vi "2025_day4.vi"() -> ()   [LabVIEW 2025]
uses:
  <userlib>/_OpenG.lib/string/string.llb/openg_string.lvlib
panel:
  out "Task 1":i16
  out "Task 2":i16
  in  "Switch":bool caption="Ex. Data  vs.  User Data"
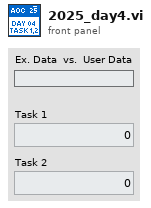
[diagram p1: front panel]
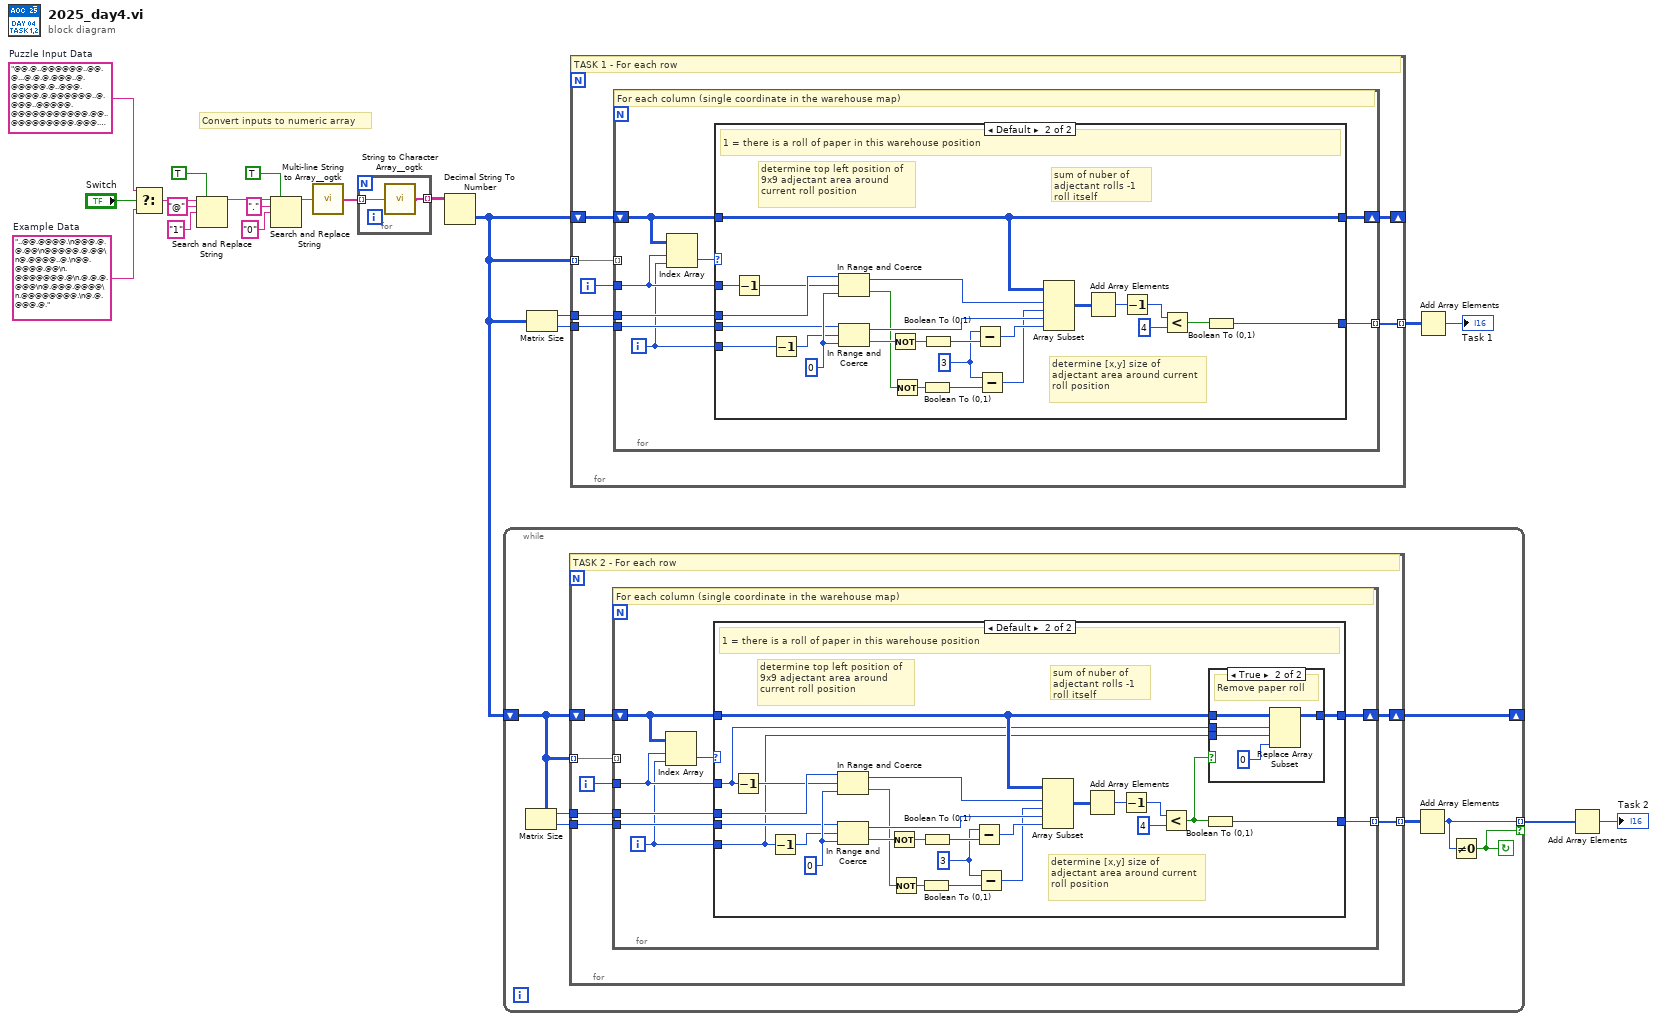
[diagram p0: block diagram]
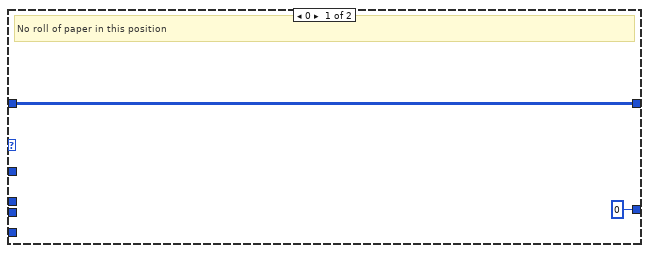
[diagram p2: hidden frame]
diagram:
  w19 = "@@.@..@@@@@@..@@.@...@.@.@.@@@..@.@@@@@.@..@@@.@@@@.@.@@@@@@..@.@@@..@@@@@.@@@@@@@@@@@.@@..@@@@@@@@@.@@@.@@@@@...@@@..@@@...@@@.@@@@@....@@@\n@.@@@.@@..@@@.@...@@..@.@@@@@@@@@@@@.@@@@....@@@.@@@@.@@.@..@@.@@@@@@@@@@@.@.@.@...@.@.@.@.@@..@.@@..@@@@@.@@@@@@..@@@@@...@..@@@@@.@..@@.@@\n@.@....@@@@.@@@@..@.@...@.@@@@@.@@@@@.@.@.@@@.@.@@@@@@@@...@@@@@@..@@..@@@@@@@@@@.@.@...@@@..@@.@@@..@@.@.@..@.@@@@@@.@@@@.@.@.@@.@@@.@@@.@@\n@@@@@@@@@@..@@.@@@@@@@@@@@@@@@@@.@@@@@....@.@......@.@.@.@..@@@.@.@@@.@...@@@@@@@@..@.@.@@..@@@@@@@@@.@@@@@@@@.@@@..@@.@.@@@@@..@@@.@@@@.@@.\n@@@.@..@@..@..@@..@@.@....@@@@..@@@@@....@.@@@.@@.@..@@@@.@@....@@.@@.@@.@@.@.@@@.@@@..@@..@.@..@@@@@@@@@@.@@@..@@.@@@.@@..@@@..@@@@@@@@.@@@\n@.@@@@@@.@@@@.@@@..@....@.@@@@@@@@@@@...@@.@@.@@@@@@..@@@@@@@...@.@@@@@@.@@@@@.@@@@@@@..@@@.@@@@@@@.@@@@@..@.@@..@@@.@.@@@@@@...@@.@@.@.@@..\n.@@@@.@.@..@@@@@.@@@@@.@@@@@.@.@@@.@@@@.@@@@@@..@@@@@@.@...@..@.@@@..@.@@.@@@@.@@.@@@..@@@..@@@@@.@@..@.@@@@.@.@@@.@..@..@@.@@@@...@@@.@@@@@\n..@.@@@@@@.@@@.@....@@@@@..@.@@@@..@@.@@@@.@..@@@@@@..@@.@@.@.@@@.@@.@@.@@@.@@@@@@.@..@@@@@@.@@@...@@@@@.@@@@@@@@....@.@@@@@@@@@@@..@@@.@@@@\n.@..@@.@@@.@@@@@.@@......@@@@@@@@.@@.@..@@..@@.@......@@..@@@@@..@@.@@...@..@@.@@@..@@.@@.@@@@@@@@@.@@@@@@.@@@.@@.@@.@...@@@@@@@.@@@@.@.@@@.\n@....@@@...@..@..@@@.@@.@@@@@@.@@@@@.@@@@.@@@@.@@@@@@@@@@..@@@@@@..@.@.@@..@.@@.@@..@.@@@.@.@.@@@@@.@.@..@@@@..@.@@..@@.@..@..@@.@....@@.@..\n@@..@@@@@@@@@@@.@.@@.@...@@@...@.@.@@@..@@.@@@@..@..@@@@@@@@@@@.@.@...@@.@@@@.@@@.@@...@@@@@.@.@.@@@.@@.@@.@.@@..@.@....@@.@.@@@@@@...@..@.@\n.@@@@..@@@@@@.@.@.@@.@@@.@@.@@.@@@@@.@.@.@.@@.@.@...@@@.@@..@.@..@@.@@.@@.@@..@@.@@@.@@.@.@@.@.@.@@@@@@@@.@..@@@@..@@.@@@.@.@.@@.@.@@..@@@@.\n@@@.@@@.@@@@@@@@@.@@@@..@@@.@@...@@.@...@@@.@.@@@...@@@.@@.@@@.@@@@@@@.@@@@.@.@@@@@@..@.@.@.@@...@@@@@@.@.@.@@@...@.@@@@@@@...@.@...@@@@@@@@\n@@@@@...@@@@.@@@..@@@@.@@@@.@.@...@.@@.@@@.@@@@.@..@@@...@.@@.@@@.@@.@.@.@@..@@@.@.@.@..@@..@.@@.@@.@..@@@.@..@.@@@@.@@@@.@@.@.@@@@@@@.@@.@@\n..@@...@@.@@.@@.@@@@@@@@@.@@.@@.@...@@@@@@@@@.@.@@@.....@@@@@@.@.@@..@..@@.......@.@@@@@@.@@@..@@@.@.@@@@@@@.@.@@..@@.@.@@@@.@@@.@@@@@@@..@@\n@@@.@@@.@@.@@..@.@.@.@@.@....@...@.@@.@@@.@@@@@..@@@@@@@@@.@@@@@@@@@@..@@...@.@@@@@@@.@@@.@@..@@@@@.@@.@..@..@@.@.@...@@.@.@@@@@@.@.@@@@@@.@\n@@@@.@@@..@@@.@.@.@@@@.@.@.@@.@@@@@@@..@@.@@@@@..@@@.@.@@@@.@@@..@@@@@@@...@@@@.@...@.@.@.@@@@@@@@@@@...@@@@@@@@@.@.@@@.@.@.@@@@@@@@@@@@@@.@\n...@@@@.@@.@@@@@@.@@@@@.@@@@@@@..@@@@@@.@...@..@@@....@@@@@@@..@@@@..@@.@@..@..@@@.@.@.@..@...@@@@@@@.@.@@@@@....@.@..@@@.@.@.@...@..@@@@@@@\n@@@@...@@...@.@.@@@@@.@@.@@..@...@@@@@@@@.@@@..@@.@@@@.@@@.@.@@..@..@@@@@@@@@...@@@.@@..@.@@@@.@@.@.@.@@@@@.@.@@@.@@@.@@@.@.@@@@@.@@@@.@@.@@\n@@.@@@.@@@@....@@@@@@@.@@@@@@.@@@@@....@.@@@@@.@@.@..@.@@.@@.@@.@@@@@@@.@@.@@...@..@.@@@.@@.@@@@.@@@@@@@.@.@.@@@@@.@.@..@@..@@@@.@@.@@@@@.@@\n@....@.@@.@@.@@..@.@@.@@@@@@@@@.@.@.@..@.@..@.@.@@.@@@@@.@@@.@..@@.@.@@@@@@@@..@@.@..@.@@@..@.@..@@@@.@@@@@@.@..@@@@@@.@@@@@...@..@.@@@...@.\n.@@@@.@@@.@.@@.@@@@@@...@@..@@.@..@@@.@.@..@@.@...@.@@@@.@@@.@..@@...@@...@@@@@@.@@.@@.....@@.@@@@@@@@@..@.@@@@@@@@.@@..@@.@.@@.@@@..@..@.@@\n@@@..@@@@......@@.@..@.@@.@@.@.@@@@@.@.....@@..@@.@@@@.@@@@@.@@.@@@@@@@@@@..@@@@@@@@@@@@@.@...@@@.@.@@@@@@@@@.@.@@@.@@.@@.@@@@.@@@@@@@@..@@@\n.@@@@@.@.@@@@@@@@.@.@@@...@@@.@@@...@@@@@.@.@.@@.@@..@@@@.@..@.@@@.@@@@@@@@@@@@.@@@..@.@.@@@@@.@@@.@@.@@.@@..@@@@@.@.@@@@.@@@@@...@@@@@@@@.@\n@.@.@@....@@@@@@.@..@@.@@.@@@@@@@@@.@@@@...@...@@..@@@@@.@@@@.@.@@.@@@@@.@@.@@....@@.@@.@@@@@@@.@@@@@.@@...@@.@@.@.@.@.@@.@@.@@.@..@@.@...@.\n@@....@..@@@@@@@@.@..@.@@.@@.@.@...@...@@..@@@@@@.@.@@.@@@@.@@.@.@@@@..@.@....@.@@..@@..@@@@@.@.@@@..@@@@@@.@@@@@@@.@.@@@@@@@@@@@@@@@@@@.@@.\n@@..@@.....@@@@@@@..@@@.....@@.@..@@@....@@@@@.@.@.@@.@..@@@@@@.@@@..@@..@@@....@.@.@@@@@...@@@@....@.@@@.@@.@@@@@.@.@..@@.@.@...@@.@..@@@@@\n@@@@..@..@.@.@@.@@@.@..@@.@@@@@@@..@@.@@..@@@.@@@@.@.@@@@@@@.@@..@@@@@@@.@@@@@@@.@@.@@..@@@@@@@@@..@..@@..@.@@.@.@.@@@@@.@@@@@@.@....@@..@@.\n@@....@@@.@.@..@@.@.@@.@.@@@...@.@@...@@@@@@.@@@@.@.@@@.@..@@@@..@@@@@@@@@@@.@@.@@@@@@@.@.@@@@.@.@@@@....@@..@@.@@..@.@@...@@..@..@.@@@@...@\n@@@@@@@@..@@.@@....@@@@.@@@.@@@@@@.@.@@..@@@@@@.@@@@.@@.@@@@.@@@.@.@@..@@@@@@@@@@@@...@..@.@..@@@.@.@@@..@@@.@.@@@@@@@@@@@@..@@@@.@.@@.@.@.@\n@@.@@@@..@@@..@.@.@.@@@.@.@@@@...@@@@@.@.@@...@@@@@..@.@@.@.@@@@.@.@@..@.@.@@@...@...@...@.@@@@@@..@@.@..@@.@.@..@@@@@@.@@@@@@@@@@@@@@@.@.@@\n@.@@@.@@@...@.@@@@@@@@@@@@..@@@@.@.@@....@@@.@.@@@@.@@..@@@.@@@@@..@.@@@@...@.@@..@@.@@.@@@@@..@@.@.....@@..@@..@@@.@.@.@@@@@@@@@.@@@..@@@.@\n..@.@@..@@..@@.@@..@.@@.@..@@..@@@@@..@@@@.@.@@.@@@@@@@.@@.@.@@@@@.@@.@@..@.@@@.@..@@@.@@.@.@@@@....@.@@@..@@..@.@@...@@@..@@..@@@@@@@@@@@.@\n@@.@@@@..@@@@@@.@@@..@.@@..@..@@@..@.@@@@@@@@..@.@@..@@@.@@...@@@.@@@@.@@.@@@@.@.@@@@.@@@.@@@@@.@@@@@.@.@@.....@@@@@..@@.@.@@@@.@@@@.@@@@@@@\n@@@@.@..@@@@@@@@..@@@..@@@@@@@@@.@@@..@@.@@.@..@@.@@@@.@@@@@@@@@@@@@..@@@..@@@@.@@@@@@@@@@@@@..@@.@.@.@..@.@.@..@.@@.@@@.@@@@.@.@@.....@....\n@.@..@@.@@@@.@@@.@@...@@.@@.@@@...@@..@@.@@@@.@..@@@@@@@@@@.@@@@@@@@@@@@@@..@.@.@.@@@@@@.@@@@...@@@@@@@@@..@@.@@.@@.@@@..@@@@@....@.@..@@@@.\n...@.@@@@@...@@@@@@@@@.@..@.@@..@.@@@@@.@.@@.@...@@@@@..@..@@@@@.@@@@@@@@@@@@....@@.@@.@@.@.@@@@.@@@@..@.@@@@@@@@@.@@@@..@@@@@@@@@@.@@@.@.@@\n@@@..@.@@@@@@@@@.@@@....@@@@@@@.@@@@@.....@@@..@@@@@.@@@@@@@@.@@@@@@.@@.@..@..@@@@@.@.@......@@@@@@@.@.@@.@@@@@@@@@.@@@@@@.@@@.@@@@.@.@.@.@.\n@..@@....@@.@.@@@@@@..@@...@@.@...@@.@.@....@@.@@@.@@...@@.@@.@.@@@@.@.@@@@@.@@.@.@@...@@.@@@@...@@@@@.@@..@.@@@@@..@@@@@@@.@@.@.@@@@@@@@@@@\n..@.@@@@@@.@.@@.@@..@@@....@.@@..@.@@.@.@@@@@@..@@@.@@.@@@.@@@@@...@@@@@.@.@@.@@@@..@.@@@.@.@@@.@@@.@@..@@@@@@@@..@@@@@@@@@..@.@.@@@@..@@@@.\n@@@@@.@.@@@@@.@@@@..@..@.@.@@@@.@@@@@@..@@@@@..@@@@...@@@..@@@.@@@.@@@@..@..@.@.@...@@@.@@@@.@...@@@.@@@....@@@@@@...@.@@@..@.@.@@@.@...@.@@\n@@@@@...@@@.@@.@@.@.@@.@@.@@@.@@@@@.@@..@@.@@@@@@@@@.@@.@@@.@@@.@@.@@.@@@@@..@.@@.@..@@...@...@@..@@.@@.@@.@@@@.@.@@@@.@@@.@@..@.@@.@..@@.@@\n..@@.@@..@....@@@..@.@.@@..@.@@.@.@@@.@@@.@.@.@@@@@...@.@@@.@@@@@..@.@@.@..@@@@.@@@@@@@@@.@@@@.@@.....@@@..@@@...@@@.@@@@@@@..@.@@@.@@@.@.@@\n..@@@@@..@@@.@.@@..@@@@@.@@@@@@@@@@.@@@@@.@@@..@..@@@.@@@.@.@@.@@@@@.@@@..@@@.@..@..@.@.@@.@.@@@@@@.@..@.@@@@@.@@@@@..@@.@@@@@..@@@@@@@.@@@@\n@.@@@.@.@@@..@@@@@...@.@@@@@.@@@@@@.@@@@..@.@@.@@.@.@@@@...@@@@@@@@.@@@@..@....@@@@@@.@.@@@..@.@.@.@@@.@.@@.@@.@@@@@..@@.@.@@@.@...@@@.@@.@@\n@@@@@..@@.@@@@@@@@@@@@@....@@@@@@@.@.@@@@.@@@@.@.@@@@@@@@.@.@@@.@@.@.@.@@.@.@..@@@@@@@@@@@@@.@...@@@@@.@@..@.@@@@@@@@.@@@.@@@@@@.@.@..@.@@@@\n@...@@.@@@@@@.@@@@@.@@@.@@@@@@.@@@@@@.@@.@...@@.@@@@..@@.@@@.@.@@@@@.@@@...@@@@@@@@@@@.@@@@.@..@..@@@@@@@@@..@@.@.@..@@@@@@@.@..@@@@..@.@.@.\n.@..@@...@.@.@@.@.@...@@@@@....@@@.@...@.@@.@@@.@..@.@..@.@.@@@.@@.@@@@@@@.@@.@.@.@@...@@@@@.@@@@@@@.@..@@.@.@.@.@..@..@@.@@.@.@.@@@.@.@@@@@\n@@@.@@@@.@@.@@@..@@.@@@@.@.@@.@.@.@@..@@@@.@.@@@@.@@..@@@...@.@@@@@@.@@@.@..@.@@@@@.@..@@...@.@@.@@@..@.@.@..@@@.@@@..@@@@@@.@@@.@@.@@@@@@@@\n@@@@..@.@@@@@@.....@@.@@@..@.@@.@.@@@@.@...@@@.@@@.@..@.@.@@@.@.@@@..@@@@@@@.@@.@@.@@@@@.@@....@@.@@.@@..@@@.@@@.@.@@@.@@@@@@@@.@@@.@....@@@\n@@@@@@.....@..@@@@@@@.@@.@@@@@.@.@@@@..@@@....@...@.@@..@@.@@...@.@.@.@@@.@.@@@@@..@.@@@@..@@@@@.@@@.@@.@@@..@@@@@..@@@.@@..@@@@.@@@...@.@@@\n@@@@@@..@.@@@@@@@@@.@@@@@.@@.@.@@@@@@@@@@@@@@.@..@@@@....@@@@.@.@.@@@.@@.@...@@@@@@@...@@@...@@.@@@@@@.@@@@@.@@...@.@@@@@@@@.@@.@@@@@@@@.@@@\n@...@.@@@.@@@@@@..@@...@@@.@..@@.@@@@@.@...@..@@@.@@@@@.@.@@@@@.@@@@@@@@@@.@@.@....@@@@@..@@@..@@@@..@@...@@@@.@@@@@.@.@..@@@@.@@.@@..@@@.@@\n@.@@..@@@.@.@.@@.@@.@@@@@@@.@@.@.@@.@@.@.@...@@@@@.@..@@@@.@..@.@@.@.@@@@...@@...@@@@.@...@.@.@@@..@@..@@@....@@@@.@..@..@@@@.@@@@@@.@.@@.@.\n@@@@.@.@@@@..@.@@....@@@..@@@@@.@@..@..@@.@@..@@.@@...@...@@@@..@@...@@@@@@@@@@..@@@.@@@.@@@@@@.@@..@@@.@@@.@@@.@.@.@@.@.@.@@.@@@@@@..@..@.@\n@@@@.@.@@.@@.@...@@@@@@@.@.@@@@...@@@.@@@@@.@@@@@.@.@@@@@@@..@@.@@..@@.@@@@@@..@@@.@@@.@....@@@@.@....@@@@@@.@.@@@@@@@.@.@@..@@@@@@@@..@@@@@\n@..@...@@@@..@.@...@@@@.@@@..@@@..@@.@@...@@@@@@@@..@@@.@@@@@@@@@@@...@...@@@@.@.@@@@@@@.@.@.@@....@@@@.@.@@@@..@.@@@..@..@.@@@.@.@...@@@.@.\n..@@@.@.@@@@.@.@@@@@@@@@@@@@.@.@@@@@@@@@@@.@@@@@@.@@@@@.@@.@@@.@@@.@@@@.@.@@.@@..@@..@.@@@.@@@@@@@.@@.@@@...@@.@@@@@...@..@@@@@@.@@@@@.@@@@@\n@@@@@@@..@@..@@.@@@.@@@.@....@@@@@.@@@.@@@@.@..@@@@.@@.@@@.@@@@@.@@@@@@@@@..@@@@@@@...@.....@@.@@@@@@@..@.@.@.@@@.@@.@@@@..@@.@@@.@.@@.@@..@\n@@.@@...@@@@@@.@@@@.@.@.@.@.@@.@...@@@@.@.@@@@....@@.@.@@@@@@@.@@@...@..@@.@..@@@.@.@.@.@.@.@@..@@@@@.@@..@@.@..@@@.@@@.@.@...@.@@@.@@@@.@@@\n.@.@.@.@@.@@.@..@@@.@.@@@.@@@...@.@...@@@...@@.@@@.@@@@@@.@.@...@...@@....@@....@.@@...@@.@@@@.@.@@@@@@@@@.@@@@@.@@@@@..@@.@@@@@.@@@@@@@.@@@\n@@@.@.@..@@@@@@@@@@@@@.@@@.@@@@@@.@@@..@.@...@@@@@.@.@@.@@.@......@.@.@@.@@@@.@@@...@@@@@@@@@@.@.@@.@.@@@@@@@@.@@@@@..@@.@@.@@@.@.@@.@.@@.@.\n@@..@@@@@.@.@.@@@@.@@.@.@@...@.@@..@@@@@@@@@@.@@@@@.@@@..@.@.@@@@@.@.@@@....@.@@.@..@..@@..@@.@@@..@@...@@.@.@@@.@@..@@@@@@@..@@@@@@.@.@.@@@\n@..@@.@.@.@@.@@@...@@.@..@@@@.@.@@@...@..@@.@.@.@@@..@@@@.@@@@@@@@.@@@@@@@..@.@@@@@@.@@@@...@@@@.@@.@@.@.@..@.@@..@.@.@@@.@@.@@@.@.@..@@@@@@\n@@..@.@.@..@.@@@@.@@@@@.@...@@@.@....@..@@@@@@@@@.@@..@.@.@@@@@@.@@..@@@@.@.@.@...@@..@@..@@@@@@@...@@@@@.@.@...@@@@...@@..@@@..@@..@@.@@..@\n@@@@....@..@@@...@@.@@@@@.@@@@.@...@@@@@@@@@@...@.@.@@@@.@@.@@@@@..@@@@@.@.@..@..@@@@.@@.@@@@@@@@.@@@@@@.....@@@@@...@.@....@@@@@@@@@@@@@..@\n@@.@@@.@@..@@.@@@..@@@.@@..@..@...@@@@@@@..@@@@@@@.@@.@@@@@.@@.@@@@.@.@@@..@@@.@..@@@@@..@.@@@@..@@@@...@@@@@@@..@..@.@@@..@.@@@@@@@@@@.@@.@\n@@@@....@@@.@@@@..@@@@@@..@@.@@.@@.@@@@@..@.@@..@..@@.@@@.@..@@@.@@@@@@.@@@.@@@..@@@@..@@@.@@@@..@@.@@@@..@@@..@@.@@@..@@@@@@@@@...@@@.@@@@@\n@@.@.@@@.@@@@..@@.@@@.@@@@.@.@@.@....@.@@@@.@@@@@@.@@@@@..@@@.@@@@@@.@@@.@@@@@@@.@@@@@@@@@@@.@.@@@.@....@.@..@.@@@..@.@...@@.@.@@@.@.@@@@@@@\n@@@@@@@.@.@@@.@@.@@.@...@@.@@.@@@@..@.@@.@@@.@..@@.@..@..@.@..@@@@@@.@.@...@@@@.@@@..@@@@..@@@.@@@@@@..@@@@@@@@.@@@@@@.@..@.@@@@@..@@@.@@@@@\n.@@.@.@@@..@@.@@.@.@@@...@@.@@@@@.@@@@@@..@@@.@.@@@.@@@....@...@@@.@.@@@.@@@@@@.@@@@..@.@.@.@.@@@@@.@@@@.@@@@.@@@...@@@@...@@.@.@@@..@@@.@@@\n...@.@.@@@.@@@@@.@@....@.@@@.@.@@.@...@@@.@.@@@@.@..@@.@@@@@@.@@@@@.@@@@@@@@.@@@@..@.@@....@@.@@@@@@..@..@@@@.@@..@.@@@@@@@@@@.@..@.@@@@@@@@\n@@.@..@@@@.@@@@@@.@@.@@@@@.@@.@.@@@..@@..@..@@.@.@@@@@.@@@@@@@@@.@@.@@..@.@@@@@@.@@@@@@.@@@.@@@.@@.@.@@.@@@@@@....@..@@@..@@@.@@@@.@@@@@@.@@\n@@@.@.@@@.@@.@.@.@@..@@@@.@.@@@.@.@...@..@..@..@.@@@.@@.@@@.@@@.@@@@@@@@@@..@@..@@.@....@@@.@.@@..@.@@.@.@@@@@@..@@.@@.@..@.@@....@.@.@@@.@@\n.@.@@.@..@..@@.@@.@@@@@@@@@@@@@..@.@@@@@@.@@@.@@@@@....@@..@@..@...@@..@.@.@@.@@@@.@@.@@@..@@@....@@@..@.@.@.@@@..@....@@.@@@@@.@@@....@@@@@\n@...@@.@..@@@@@@..@@@@.@@@...@@@..@@@.@@.@@@@.@..@@@@..@..@.....@@@.@@@.@@..@..@@@@.@.@@.@@.@@@@.@@.@.@.@...@@@.@@@.@..@@.@@..@@@.@...@@@@@@\n@.@@@.@@@.@...@@@@@@@@@@.@@@@@@.@.@..@....@@@...@@@.@@@@@..@@.@....@..@@.@.@..@@@@.@@@.@.@@@@@@@.@@@@@@@@@.@@@@@@.@@@@@@@.@..@@@@@@@@.@@..@.\n@@..@@@@.@@@@@.@@@.@.@@@.@@.@.@.@@@@@@@...@...@.@.@@.@@@@@@@.@.@...@@@@@@.@@.@@...@@@..@@@@@@@.@.@.@@..@....@@.@@.@@@@.@@@@@@@..@.@@....@.@.\n.@..@.@..@@@@...@..@@@.@@.@@@.@@@@.@.@@@@@@.@@@@@@@..@@@@.@..@@@.@@.@.@.@@.@@@@.@@@.@@.....@.@@@@@.@....@@@.....@@.@..@@@.@@@.@@..@.@@@@.@@.\n@@.@.@...@....@.@..@@.@@..@.@.@@@@.@.@@...@@@.@.@.@@..@@@.@@.@@.@@@.@@@@@...@@.@@@.@..@..@..@@@@@..@@@.@@..@@.@@@@..@@@.@@@@.@.@.@@.@@@@@@..\n.@@.@@.@.@..@..@@..@.@@.....@@@@@.@@@@@@.@..@..@@@@.@.@.@@@.@.@.@.@.@@...@@.@@.@.@@.@@@.@@@@@@.@.@@@@@@@@@.@.@@@@@..@@@@@.@.@@@@@.@...@@....\n@...@.@@@@.@@@@.@@@.@.@@@..@@@@...@@@.@@@@@@@.@@@.@.@@@.@@@.@@..@..@.@.@@@@.@@@.@.@@.@@...@...@@@@@@@.@@@@@.@@.@@@..@@@..@@@@@@@@@@..@.@.@.@\n@@@@..@.@.@@@..@@@@@..@@@@@..@@@@..@.@@.@@.....@..@@.@.@@...@@@.@.@..@@..@@@@.@..@@@@@@@@@@.@...@@.@@....@.@@@@@@...@.@.@@..@@@@.@.@@@@...@@\n.@@@@..@@.@@..@@..@..@.@..@@.@@.@.@@@.@.@..@.@...@.@.@@@@...@@@.@@..@.@.@@@@@@@@.....@@@@.@@@.@...@@@@@.@@.@@.@@....@@@@.@.@@@.@@@@..@@@@@@@\n.@......@@@@@@...@.@.@..@..@@.@@.@@@@@.@@@@@@@.@@@@@@.@@@.@.@.@@.@@.@@@.@@..@@@@@.@@@@@@.@.@.@.@@.@@@.@@..@.@.@.@...@.@.@.@......@.@.@.@@@.@\n@@@@@..@@@.@@@@@.@.@@@.@@@@@@@@@@@@@.@@..@@@@@.@@.@@..@@@@@@@@@@..@@@@@.@@.@@@.@@..@@..@.@@.@@@.@@@@.@.@.@....@@@@.@@@@@@@@@@@@@@@..@.@@.@.@\n.@.@@@@@.@@@@@@@@@@@@@@@@.@..@.@@@@.@@..@@@@..@.@.@.@.@.@.@@@@@@.@...@@@@@...@...@@.@@@@@@@@@@@@@.@@..@@@@@@@@@.@@.@.@@@@@@@@@@@@@@@@@@@@@@.\n@@..@.@@@.@@@@.@@@.@@..@.@@@@@@@...@@@@@.@@@@.@.@@@@@@..@@@@.@@@@@@@@...@@@...@@...@@.@.@@@.@..@@.@@@@.@@@...@@..@@@@@@@@..@@...@..@@.@@@..@\n@@..@@@...@.@@@@@@@@@.@..@@@.@.@@.@@..@@.@.@.@.@@..@@@@.@..@..@.@@@@@@.@.@..@@@@.@.@@.@.@@@...@.@@@@@@@.@..@@@@.@@@.@@.@@@@.@@.@.@.@@.@@@@@@\n.@@.@.@@.@@..@@@@@..@@.@@..@..@.@...@@.@@@@@.@.@@@@@@.@..@@.@@@@@@@@@.@@@@@..@...@.@.@@@@@....@@@@@@@@@.@@.@@.@@.@.@@.@@..@@@@..@@@.@@@@.@@@\n.@..@@@.@.@@.@@@@...@.@@@@@.@@@@.@.@.@@@.@.@@@@.@.@@@..@.....@@.@@@@@@.@@@.@@.@.@@@@@@@@@@..@..@@@@..@@.@@@@@.@..@@@@@@@@.@@.@.@.@@@@@@..@.@\n@@@@@.@.@@@@@@@@@@@.@@@.@@...@...@@@@@.@...@@@@@.@@@@..@@@@@.@...@.@@@@@.@@@@.@@@@.@@@.@@...@@@..@@.@@@.@.@@@@.@@@@@.@@@@.@@@@@.@@@@@@@@@@.@\n@@@@@@.@.@..@@@.@..@.@.@.@@.@..@..@@@@@@.@.@.@@...@@..@@@@@.@@......@.@@@@@@.@@@.@@.@.@@@@...@.@..@@@@..@@@.@@@.@.@.@@@@@@@@@@@.@@@.@@.@.@@@\n@.@...@.@@@.@..@.@@..@@.@.@.@@@.@@@...@@@.@@.@@@.@@@.@.@@@.@@@.@..@@..@.@.@@@@@@@..@@@@@@@@..@.@@@@@..@.@@@@@@@@@....@@@@@@..@.@.@.@@@.@@...\n@.@@@@@.@@@.@@@@..@@.@@.@@@.@@@@@.@@@.@.@@@@.@@@@@@@@....@@.@@@.@..@@.@@@.@@@.@.@@@..@.@..@@@.@@@@..@.....@@.@@@@.@@...@@@@..@@..@..@@@..@@@\n@@@@@..@.@.@.@@@@.@@...@@@@@@@..@..@@@@@@@.@@@@..@@.@@@@.@@@@....@@.@@.....@.@@....@@.@@@@@@.@.....@.@.@@@..@@.....@@@..@@@.@@..@@@@@.@.@.@.\n@@.@..@@@.@.@@@@@@.@@@@@@.@@@...@@@@@@..@@@..@@@@@@@.@.@@@@.@@@.@@@@@@.@@@@@@@.@..@.@@@@@.@@.@@@..@.@@.@@@...@@.@@@.@@.@@@@.@@@@@@@.@.@.@..@\n.@.@..@@@...@@@.@@@@@..@@@.@..@..@@@@.@@@.@@@@@.@@@..@@@@.@.@@.@@@@..@..@.@.@@@@.@.@.@@@@@@@@@.@@@@@.@.@.@@.@@@.@@.@....@.@@@..@@.@@..@.@...\n.@@@@@.@@@..@@.@.@@.@.@@@@@@@..@@..@.@.@@@.@@@@@@@@.@@..@@@...@@@@@..@@.@@@@.@@.@.@@@.@..@@.@@..@....@@.@@@@.@.@@@.@.@.@.@@@.@@.@@.@@@.@..@@\n@@....@@@@@.@@.@..@@@@.@@.@.@@@...@.@...@..@@..@@.@@@@@.@.@..@...@.@@@@@@.@@..@.@.@.@@.@@@..@@@.@@.@..@@@.@@@@@.@@.@..@.@@@.@.@..@@.@@@@.@@.\n@@@@.@@@..@.@.@..@@@@@@.@@..@@.@.@@.@..@@@@..@@.@.@@.@@..@.@...@.@.@@@@@@.@@@@@@.@.@@@.....@@.@@@@@@@.@@@@.@@@@@@@@@@@@@@@.@.@.@@@@@@@.@@@@.\n.@@@..@@@....@@@@@@@.@@@@@@.@@..@@..@@@@.@@@@....@@...@.@.@@@@@.@@@..@.@.@@@@.@@@@..@.@.@@.@@.@@...@..@.@@@..@@...@.@.@@...@.@..@@@@@@@.@.@.\n@.@@@@.@@.@.@@@.@.@.@@@.@@@.@.@@..@@@@@@@@@@@@@@.@@@@@@@@.....@@@@@.@@@@@@@@@...@@.@..@.@@@@@.@..@@@..@.@@.@@@.@@.@.@@@@@@@@@@@....@@@@@@.@@\n@@.@@@@@@.@@@.@.@@.@@@@.@@...@@@@@@@.@@.@.@@@.@@@@@@..@@@@@..@.@.@@@@.@@@..@@@@@@.@@@@@@@..@@.@@.@@@@....@@@..@@@@..@@.@@@..@@@...@@@@.@@@..\n.@@@.@.@.@..@@@@@@@.@.@.@@..@.@.@.@@@@.@..@.@@@....@@@.@@@.@.@@@@@...@.@@@.@@@..@.@@@...@@@@@@..@@.@.@.@@@.@@@@.@@@.@@@@@..@@.@@@@@@.@@@.@@@\n@@.@....@.@@@@@@..@@...@@@@@@@@@@@@@@@@@.@@@.@@..@.@.@@@@@.@@.@.@@@..@..@@@.@@@@@.@.@@@@@@@.@@.@@.@@.@@@.@.@@..@@@.@@@.@@.@@@...@@@@@@@.@@@.\n@..@@@.@@.@@@@@...@....@@.@@.@@@@@@@@@..@...@@@@...@.@@@.@.@.@@.@@@@@@@@.@@@@@@@@.@@.@@.@.@@@.@.@@@.@@@@@.@.@.@@@@@..@@@@@..@.@.@@@@@@@@@.@@\n@@..@@@@@@@@@@@...@@@@@@@@@@@@@.@...@@.@@@..@@@@@@@@@@@@@@..@@@@@..@@.@@@@@@......@@@@.@@@.@@.@@@@..@.@@..@@..@..@.@@.@@@.@@.@@@@@@@@..@.@@@\n@@.@.@@@@@.@..@@.@@@...@@..@@.@..@@@.@@@.@....@@...@@.@@@@.@.@.@@@@.@@@.@.....@.@.@@@@@.@.@@@..@@@@@.@@@...@@@@..@@.@@.@@.@@.@@.@...@@@@.@@@\n@@.@.@@@.@@..@@..@@.@.@@@.@@@@@.@.@@..@.@..@...@@@@@@@...@..@@@@@@@@@@@...@@.@@.@@@@.@.@@@@@@@@.@.@@.@@.@@@...@@.@...@@@@...@@@@@.@@.@@@@.@@\n@@@@@.@@@.....@...@@.@@@@.@.@.@.@.@.@@.@..@.@@@@.@@.@@@@@.@.@@@.@@@..@@...@@@@@.@@.@@@@@@@@@@@@@.@@.@@@.@.@.@.@@@.@.@.@@@@@@@@@.@.@@@@.@@@@@\n@.@@..@@@.@.@.@@.@@@@..@@@@@.@.@@.@@@.@@@.@....@@@..@.@.@@@..@@.@@@.@@@@@@@...@.@@@@@....@@@.@@...@.@.@..@@@..@@.@.@@.@....@@@@@@@@@@.@@@..@\n....@.@@@@.@@@@@.@..@@.@.@.@@@@@.@@@@.@@@...@@.@.@@@@.@.@@@..@.@@.@@.@@.@@.@@@@@..@@@.@@@..@@.....@.@@@@@..@@.@.@...@@.@.@@.@..@@@@@@@.@@@@.\n@@@@.@@@.@@.@@@@@.....@@@@@@..@@.@@@..@@@.@.@@@@..@@.@.@.@@@@@@..@..@@@@.@@@@@@..@.@@@@@@@..@@@@...@@@@....@@.@@@..@@.@..@@@@@@@@@@@@@@@@@..\n@.@@@@.@@.@@@..@@@...@@@@@@@@..@@@.@@@@@@....@@.@@.@@@.@@@@@@@@@@@@@@@.@.@@.@@.@@.@...@@@@.@@.@.@@@....@.@@@@@.@@@@..@@@@..@.@..@..@@@.@@@.@\n@..@.@......@@...@@....@@@.@@@..@@..@.@.@@....@.@@..@@@@.@@@@.@@@@@@@.@.@.@@..@@@.@@.@.@...@@.@@@@@@@..@@.@@@@..@@@@..@@@@.@.@@@.@@..@@.@@..\n@....@.@.@@@.@@..@...@@@@@@.@@..@.@@.@.@@@@@@@@@@@..@@@.@@@..@@@@@.@@@@.@..@@.@@@@.@@@@@.@...@@@@@@@@@@..@@@@.@.@.@@.@@@@.@@@@@@@...@.@.@.@@\n@@.@.@.@@.@@..@..@@@@@@@..@.@@@@@.@.@@.@@@..@@.@@@@@@@.@@.@@.@@.@@@@@.@@@..@@..@.@.@@..@@.@.@@@.@.@@@.@@@.@@@@@.@@@.@@@@@....@.@@....@.@@@@@\n.@...@.@@@.@@@@@@.@.@@.@@@@@.@..@@@@@@@.@@.@@@@.@.@@@@..@..@@@@.@@@@@.@.@.@@@@@....@.@@.@@@.@@@@@.@@.@@@.@@@.@.@@@.@..@@.@...@@@@@@@@@.@@@@@\n@@..@.@@...@@@@@@@@@@@..@.@.@.@@..@.@.@.@.@@..@@.@@@@@@@@@@.@@.@@@@@@@@.@@@@@.@@.@@@.@@@.@@@.@@@@.@...@@@@...@@@@@@.@..@@@..@..@.@@..@....@.\n..@.@.@@...@@..@.@@@@@@@@@..@@@@..@.@@@@@@@.@.@..@@@.@.@@@@.@..@@.@@..@.@.@@...@@@..@@@@...@..@..@@.@..@@@@@..@@.@@...@@.@@@.@@.@..@..@@@@@@\n@@..@@.@.@@@@@@..@.@@.@.@@@...@..@@@@@.@@@@..@@@@.@@@@@@@@.@.@@@.@@@@@@.@.@@@@.@.@...@@.@@@..@......@@.@@...@@@@.@..@.@@@@@@@.@@......@.@.@@\n@.@..@@@@@.@@@@@@@.@.@@@@@.@..@.@@...@@@@@..@@@@@@..@@....@@.@@@@@@.@@.@.@..@@@@@@.@@.@.@.@@@@..@.@.@@@@@.@@@..@@.@@..@...@@@@@...@@.@.@@@@@\n.@@@.@.@@@@.@@@..@@@@@..@@.@@.@..@.@@@@@.@@.@...@....@.@..@..@@.@@@@@@@.@@@@.@.@@@.@@@@@@@@@@@@.@.@@@@@@@@@.@.@.@@.@.@@@@@@.@..@@@@@...@@..@\n@.@.@@@@@..@...@.@@@@@.@@.@..@@...@@.@@@@.@..@@@.@.@@..@.@@.@.@..@.@.@@@..@@.@@.@@..@.@@..@@.@@..@.@.@@@@.@.@@@.@.@.@@@@@@.@.@@@.@@@.@@.@@@@\n@@..@.@@@..@@@@@.@@.@.@.@@@@@..@...@.@@@.@@.@@@@.@@@@@@@@@..@@@@@@@@...@@...@@@.@@@.@@.@.@@...@.@.@.@.@@@.@@@@@.@@@.@@@@..@@@@@..@.@@@.@@@@@\n...@@..@.@@@@@@@@@@.@@.@@@.@@..@@.@@@@@..@@@@@@@..@.@@..@@@.@@@@.@@@@@@@...@..@@..@@@@.@.@...@@.@@@@@@.@.@..@.@@@.@@@.@@@@@@.@.@@..@@@@@@@@@\n@@@@.@..@@@@@@@@.@.@.@@@.@@...@@@@@@@@@.@..@@@@@@@@@@@@@@..@@@@@@@.@.@...@..@@@.@@...@.@..@@@.@@@@..@.@@@@@....@.@@@..@@@@@@@@...@@@@.@.@@@@\n@@@@@@.@@@@@..@@@@.@@@@.@@..@@@@@@.@@@@@...@...@@@.@.@@@@.@@@.@@..@@.@..@@@@@@@@@@@@.@@@.@.@@@.@@.@@.@..@@@.@@@@@@@@@@.@.@@@@@@.@@@@.@@@@@@.\n.@.@@@@@@@@@@@@@@.@@.@@@.@@.@@.@@@.@....@@@@@.@.@@@@...@@@.@@.@@@@..@@.@@.@@.@.@@@.@.@@@.@.@@@@@@@@@.@@@....@@.@@@@@@.@.@@@.@@...@@.@.@.@@@@\n.@.@@@.@@@@@@@@.@@@.@@@@...@@@@@@@@..@@@.@@@@@@.@.@@@@.@.@@..@@@@@@.@....@.@@@@@@@..@@@.@@@@@@@@.@@...@@@@@.@@.@@.@@@@@@@@...@.@@@@@@..@@@@@\n@@.@..@@.@@@@@.@@@@@.@@@@@@@@@@@@@@..@@@.@@.@.@@.@@@@.@@@@@@@@@@@.@.@@@@...@.@.@@@@@.@.@.@...@@@.@.@@@@@..@@@@@@@@@..@.@@.....@@@@@@.@.@.@@@\n@.@..@.@.@.@@@@@..@@@@..@@@@@@.@.@@.@@@.@@@@.@@@@@@@@@@@...@@.@@.@@.@@@@@@@.@@.@@@.@@@@@...@@.@@..@.@@@.@@.@..@@.@@.@@@@..@@@.@@@@@.@@@@@@.@\n@@.@@.@@.@@@@@@@@@@@@@.@.@@@.@@.@.@@@@.@@@..@@@@.@@@.@@@.@@@@@@@@@..@@.@....@@@@@.@.@@@.@@...@@@..@@@@@..@.@@@@@.@@@@.@@@@.@@@.@@@@@@...@@@.\n....@@...@@.@@@@@@...@..@@.@..@.@...@..@@@@@@.@@@@@@@@@@..@..@@.@.@.@@@.@@@@@@.@@.@...@.@..@.@@@@.@.@.@@@@@@@@.@@@@@.@@@..@@@.@@@@.@@@@.@@@.\n@.@@@@@.@@.@.@@@@@@@@@..@@.@@@.@@@@@@@.@@.@@..@@..@@.@@@.@@@@@.@@@@@.@@..@.@...@.@@@@@....@.@@.@@@@@@@@@@@@@.@.@@.@.@..@@@@@@.@@@.@.@.@@@@@@\n...@@.@@@@@@@....@.@@@@.@..@@....@@.@.@@.@@@.@@@@@@.@.@@@@@.@@..@@@.@@.@..@..@@.@@.@@..@@@@@@.@@@.@@@@.@@@@.@@@....@.@@@.@@.@@..@.@@@@@@.@@@\n.@@@.@@@...@@.@@@@@..@.@@@@@@@@@.@.@@@.@@@@@@@@@@.@.@@@@.@@@@@..@...@@.@@..@@.@.@@@@@@@.@@@@@@@@@@@.@@@@@@..@@.....@@.@@@@.@@@..@@@@...@@@@.\n@.@@@@..@@.@@@@@.@.@..@.@.@@..@@..@@@@.@@@@@..@@@@..@@@..@@@@.@@@@@..@..@@....@@@.@.@@@.@.@@@...@@@@@@@@@@@.@@@@@.@.@@..@@.@@..@@@.@.@@@@@.@\n@@.@@@@@.@...@@@@@@@.@@@.@@@....@@@@@@@..@@@.@@.@.....@.@@@@@@.@.@.@@@@....@@.@@@..@@@@...@.@@@@@@@@.@@@.@@.@..@.@@@@@@@.@.@.@@@@@..@@.@.@@."  # Puzzle Input Data
  w20 = "..@@.@@@@.\n@@@.@.@.@@\n@@@@@.@.@@\n@.@@@@..@.\n@@.@@@@.@@\n.@@@@@@@.@\n.@.@.@.@@@\n@.@@@.@@@@\n.@@@@@@@@.\n@.@.@@@.@."  # Example Data
  # "Convert inputs to numeric array"
  n1 = Select(t=w19, s="Switch", f=w20) -> (s? t:f=w17:string)
  n2 = Search and Replace String(replace all?=TRUE ("replace all? (F)"), input string=w17, search string="@", replace string="1" ("replace string (\"\")")) -> (result string=w11:string)  [unwired: 4 in, 3 out]
  n3 = Search and Replace String(replace all?=TRUE ("replace all? (F)"), input string=w11, search string=".", replace string="0" ("replace string (\"\")")) -> (result string=w10:string)  [unwired: 4 in, 3 out]
  n4 = call <userlib>:"Multi-line String to Array__ogtk.vi"("string"=w10) -> ("lines"=w9:string[])
  n5 = for {
    tunnel: w9 -> [w23] mode=indexing
    tunnel: [w22] -> w8 mode=indexing
    n6 = call <userlib>:"String to Character Array__ogtk.vi"("Input String"=w23) -> ("Character Array"=w22:string[])
  }
  n7 = Decimal String To Number(string=w8) -> (number=w2:i32[][])  [unwired: 2 in, 1 out]
  n8 = while {
    tunnel: [w26] -> w7 mode=indexing if=w25
    shift-right: [w27] -> _
    shift-left: w2 -> [w24]
    stop <- w25 continue-if-true
    n9 = Matrix Size(0:w24) -> (1:w30:i32, 2:w29:i32)
    n10 = for {
      tunnel: w24 -> [w35] mode=indexing
      shift-right: [w36] -> w27
      shift-left: w24 -> [w37]
      tunnel: w30 -> [w33]
      tunnel: w29 -> [w32]
      tunnel: [w31] -> w28 mode=indexing
      i -> [w34]
      # "TASK 2 - For each row"
      n11 = for {
        shift-right: [w40] -> w36
        shift-left: w37 -> [w41]
        tunnel: w35 -> [_] mode=indexing
        tunnel: w34 -> [w39]
        tunnel: w33 -> [w45]
        tunnel: w32 -> [w44]
        tunnel: [w42] -> w31 mode=indexing
        i -> [w38]
        # "For each column (single coordinate in the warehouse map)"
        n12 = Index Array(array=w41, index (row)=w39, index (col)=w38) -> (element=w43:i32)
        n13 = case shown="Default" w43 {
          tunnel: w45 -> [_ w72]
          tunnel: w44 -> [_ w69]
          tunnel: w41 -> [w46 w53]
          tunnel: [_ w54] -> w42
          tunnel: [w46 w52] -> w40
          tunnel: w39 -> [_ w50]
          tunnel: w38 -> [_ w48]
          frame 0 {
            # "No roll of paper in this position"
          }
          frame Default {
            w60 = 3 ("y")
            w71 = 0 ("lower limit")
            # "sum of nuber of adjectant rolls -1 roll itself"
            # "determine [x,y] size of adjectant area around current roll position"
            # "determine top left position of 9x9 adjectant area around current roll position"
            # "1 = there is a roll of paper in this warehouse position"
            n14 = Decrement(x=w50) -> (x-1=w51:i32)
            n15 = Decrement(x=w48) -> (x-1=w49:i32)
            n16 = In Range and Coerce(upper limit=w72, x=w51, lower limit=w71) -> (coerced(x)=w68:i32, In Range?=w61:bool)
            n17 = In Range and Coerce(upper limit=w69, x=w49, lower limit=w71) -> (coerced(x)=w70:i32, In Range?=w67:bool)
            n18 = Not(x=w67) -> (.not. x?=w66:bool)
            n19 = Not(x=w61) -> (.not. x?=w62:bool)
            n20 = Boolean To (0,1)(Boolean=w62) -> (0, 1=w63:i16)
            n21 = Boolean To (0,1)(Boolean=w66) -> (0, 1=w65:i16)
            n22 = Subtract(x=w60, y=w65) -> (x-y=w64:i32)
            n23 = Subtract(x=w60, y=w63) -> (x-y=w59:i32)
            n24 = Array Subset(array=w53, index (row)=w68, length (row)=w59, index (col)=w70, length (col)=w64) -> (w58:i32[][])
            n25 = Add Array Elements(numeric array=w58) -> (sum=w56:i32)
            n26 = Decrement(x=w56) -> (x-1=w55:i32)
            n27 = Less?(x=w55, y=4) -> (x < y?=w47:bool)
            n28 = Boolean To (0,1)(Boolean=w47) -> (0, 1=w54:i16)
            n29 = case shown="True" w47 {
              tunnel: w53 -> [w73 w78]
              tunnel: [w73 w77] -> w52
              tunnel: w50 -> [_ w76]
              tunnel: w48 -> [_ w75]
              frame False {
              }
              frame True {
                # "Remove paper roll"
                n30 = Replace Array Subset(array=w78, new element=0 ("new element/subarray"), index (row)=w76, index (col)=w75) -> (w77:i32[][])
              }
            }
          }
        }
      }
    }
    n31 = Add Array Elements(numeric array=w28) -> (sum=w26:i16)
    n32 = Not Equal To 0?(x=w26) -> (x != 0?=w25:bool)
  }
  n33 = Matrix Size(0:w2) -> (1:w5:i32, 2:w4:i32)
  n34 = for {
    tunnel: w2 -> [w83] mode=indexing
    shift-right: [w84] -> _
    shift-left: w2 -> [w85]
    tunnel: w5 -> [w81]
    tunnel: w4 -> [w80]
    tunnel: [w79] -> w3 mode=indexing
    i -> [w82]
    # "TASK 1 - For each row"
    n35 = for {
      shift-right: [w88] -> w84
      shift-left: w85 -> [w89]
      tunnel: w83 -> [_] mode=indexing
      tunnel: w82 -> [w87]
      tunnel: w81 -> [w93]
      tunnel: w80 -> [w92]
      tunnel: [w90] -> w79 mode=indexing
      i -> [w86]
      # "For each column (single coordinate in the warehouse map)"
      n36 = Index Array(array=w89, index (row)=w87, index (col)=w86) -> (element=w91:i32)
      n37 = case shown="Default" w91 {
        tunnel: w93 -> [_ w120]
        tunnel: w92 -> [_ w117]
        tunnel: w89 -> [w95 w96]
        tunnel: [i16 0 w102] -> w90
        tunnel: [w95 w96] -> w88
        tunnel: w87 -> [_ w100]
        tunnel: w86 -> [_ w98]
        frame 0 {
          # "No roll of paper in this position"
        }
        frame Default {
          w108 = 3 ("y")
          w119 = 0 ("lower limit")
          # "sum of nuber of adjectant rolls -1 roll itself"
          # "determine [x,y] size of adjectant area around current roll position"
          # "determine top left position of 9x9 adjectant area around current roll position"
          # "1 = there is a roll of paper in this warehouse position"
          n38 = Decrement(x=w100) -> (x-1=w101:i32)
          n39 = Decrement(x=w98) -> (x-1=w99:i32)
          n40 = In Range and Coerce(upper limit=w120, x=w101, lower limit=w119) -> (coerced(x)=w116:i32, In Range?=w109:bool)
          n41 = In Range and Coerce(upper limit=w117, x=w99, lower limit=w119) -> (coerced(x)=w118:i32, In Range?=w115:bool)
          n42 = Not(x=w115) -> (.not. x?=w114:bool)
          n43 = Not(x=w109) -> (.not. x?=w110:bool)
          n44 = Boolean To (0,1)(Boolean=w110) -> (0, 1=w111:i16)
          n45 = Boolean To (0,1)(Boolean=w114) -> (0, 1=w113:i16)
          n46 = Subtract(x=w108, y=w113) -> (x-y=w112:i32)
          n47 = Subtract(x=w108, y=w111) -> (x-y=w107:i32)
          n48 = Array Subset(array=w96, index (row)=w116, length (row)=w107, index (col)=w118, length (col)=w112) -> (w106:i32[][])
          n49 = Add Array Elements(numeric array=w106) -> (sum=w104:i32)
          n50 = Decrement(x=w104) -> (x-1=w103:i32)
          n51 = Less?(x=w103, y=4) -> (x < y?=w97:bool)
          n52 = Boolean To (0,1)(Boolean=w97) -> (0, 1=w102:i16)
        }
      }
    }
  }
  n53 = Add Array Elements(numeric array=w3) -> (sum=→"Task 1":i16)
  n54 = Add Array Elements(numeric array=w7) -> (sum=→"Task 2":i16)
